vi "Prepare Execution.vi"(7 "Options (Default)":T1={"Use Default Model (T)"=TRUE, "Release Related References (T)"=TRUE}, 8 "error in (no error)":errorcluster, 11 "Engine in":refnum<class "Engine.lvclass">) -> (0 "error out":errorcluster, 2 "Execution":refnum<class "Execution.lvclass">, 3 "Engine out":refnum<class "Engine.lvclass">)   [LabVIEW 2020, in "TSnax.lvlib" / "Engine.lvclass"]
uses:
  Engine.lvclass
  Engine.lvclass/Engine.ctl
  Execution/Execution.lvclass
  Execution Response.ctl
  Execution Options.ctl
  TSnax.lvlib
  New Execution Request.ctl
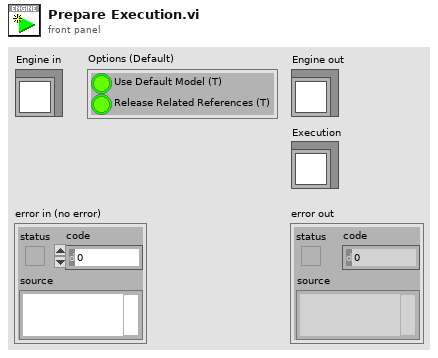
[diagram p1: front panel]
types:
  T1 = typedef "TSnax.lvlib/Execution Options.ctl" = cluster{"Use Default Model (T)":bool, "Release Related References (T)":bool}
  T2 = typedef "TSnax.lvlib/Engine.lvclass/New Execution Request.ctl" = cluster{"Options":T1, "Notifier":refnum<notifier>}
  T3 = typedef "TSnax.lvlib/Engine.lvclass/Execution Response.ctl" = cluster{"Execution":refnum<class "Execution.lvclass">, "Error":errorcluster}
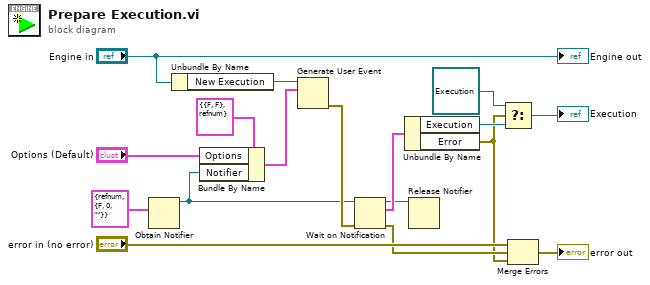
[diagram p0: block diagram]
diagram:
  n1 = Obtain Notifier(notification data type=T3 {"Execution"=refnum, "Error"={"status"=FALSE, "code"=0, "source"=""}} ("Execution Response")) -> (notifier out=w9:refnum<notifier>)  [unwired: 3 in, 2 out]
  n2 = Unbundle By Name("Engine in") -> ("New Execution"=w11:refnum<user-event>)
  n3 = Bundle By Name(cluster=T2 {"Options"={"Use Default Model (T)"=FALSE, "Release Related References (T)"=FALSE}, "Notifier"=refnum} ("New Execution Request"), "Options"="Options (Default)", "Notifier"=w9) -> (w10:T2)
  n4 = Generate User Event(user event=w11, event data cluster=w10) -> (error out=w17:errorcluster)  [unwired: 2 in, 1 out]
  n5 = Wait on Notification(notifier=w9, error in (no error)=w17) -> (notifier out=w7:refnum<notifier>, notification=w8:T3, error out=w5:errorcluster)  [unwired: 2 in, 1 out]
  n6 = Unbundle By Name(w8) -> ("Execution"=w4:refnum<class "Execution.lvclass">, "Error"=w3:errorcluster)
  n7 = Release Notifier(notifier=w7) -> ()  [unwired: 2 in, 3 out]
  n8 = Select(t=refnum<class "Execution.lvclass"> refnum, s=w3, f=w4) -> (s? t:f=→"Execution":refnum<class "Execution.lvclass">)
  n9 = Merge Errors("error in (no error)", w5, w3) -> (→"error out":errorcluster)
  "Engine out" <- "Engine in"
